vi "GetDiskFreeSpace.vi"(0 "RootPathName (C:\\)":string="c:\\", 11 "error in (no error)":errorcluster) -> (1 "TotalBytes":u32, 2 "Free Bytes":u32, 3 "TotalNumberOfClusters":u32, 4 "Dup RootPathName (C:\\)":string="c:\\", 12 "SectorsPerCluster":u32, 13 "BytesPerSector":u32, 14 "NumberOfFreeClusters":u32, 15 "error out":errorcluster)   [LabVIEW 2011, in "API.lvlib"]
doc: "Retrieves information about cluster sizes, sector sizes, free and used space on the requested drive."
uses:
  API.lvlib
  kernel32.dll
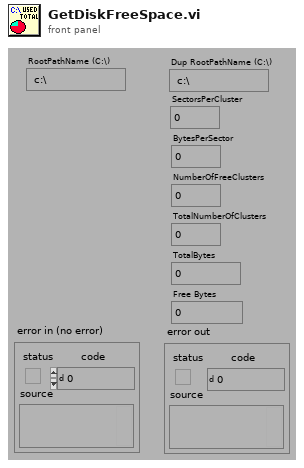
[diagram p1: front panel]
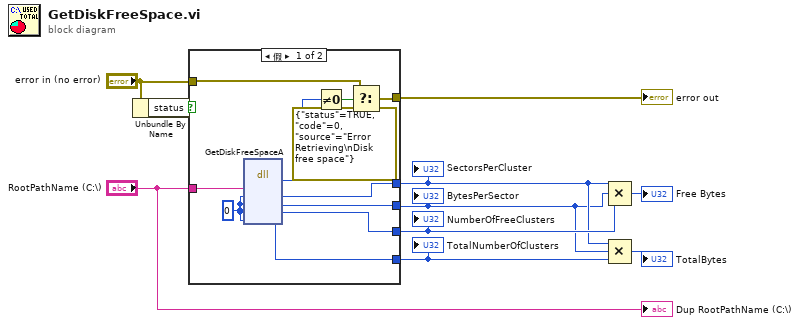
[diagram p0: block diagram]
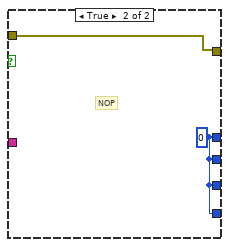
[diagram p2: hidden frame]
diagram:
  n1 = Unbundle By Name("error in (no error)") -> ("status"=w7:bool)
  n2 = case shown="假" w7 {
    tunnel: "RootPathName (C:\\)" -> [w20 _]
    tunnel: [w19 w23] -> w4
    tunnel: [w18 w23] -> w3
    tunnel: [w17 w23] -> w10
    tunnel: [w16 w23] -> w9
    tunnel: "error in (no error)" -> [w13 w22]
    tunnel: [w12 w22] -> w6
    frame False {
      w21 = u32 0 ("lpSectorsPerCluster")
      n3 = dll-call lib="kernel32.dll" fn="GetDiskFreeSpaceA" label="Get Disk Free Space"("lpRootPathName"=w20, "lpSectorsPerCluster"=w21, "lpBytesPerSector"=w21, "lpNumberOfFreeClusters"=w21, "lptotalNumberOfClusters"=w21) -> (w15:u8, "lpSectorsPerCluster"=w19:u32, "lpBytesPerSector"=w18:u32, "lpNumberOfFreeClusters"=w17:u32, "lptotalNumberOfClusters"=w16:u32)  [unwired: 4 in, 2 out]
      n4 = Not Equal To 0?(x=w15) -> (x != 0?=w14:bool)
      n5 = Select(t=w13, s=w14, f=errorcluster {"status"=TRUE, "code"=0, "source"="Error Retrieving\nDisk free space"}) -> (s? t:f=w12:errorcluster)
    }
    frame True {
      w23 = u32 0 ("lpSectorsPerCluster")
      # "NOP"
    }
  }
  "SectorsPerCluster" <- w4
  "BytesPerSector" <- w3
  "NumberOfFreeClusters" <- w10
  "TotalNumberOfClusters" <- w9
  "error out" <- w6
  n6 = Compound Arithmetic op=MULTIPLY(w4, w3, w10) -> (→"Free Bytes":u32)
  n7 = Compound Arithmetic op=MULTIPLY(w4, w3, w9) -> (→"TotalBytes":u32)
  "Dup RootPathName (C:\\)" <- "RootPathName (C:\\)"
